vi "Default controls - save controls values.vi"(8 "error in (no error)":errorcluster) -> (0 "error out":errorcluster, 2 "VI's path in related to the INI":path, 3 "INI's path to the saved controls":path)   [LabVIEW 2020]
uses:
  Save-Load-Defaults.lvlib/Save-Load-Defaults.lvlib
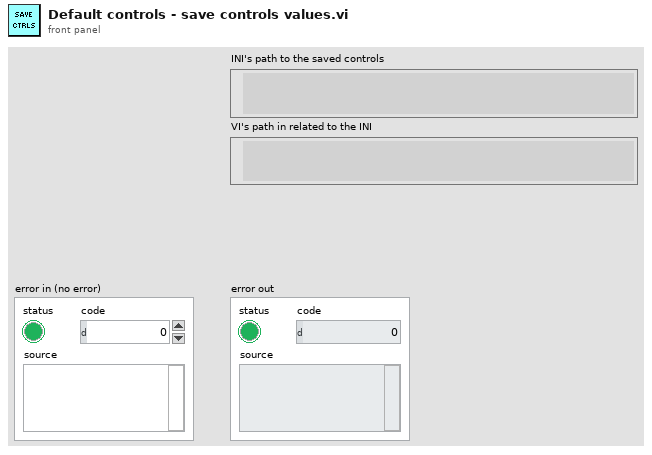
[diagram p1: front panel]
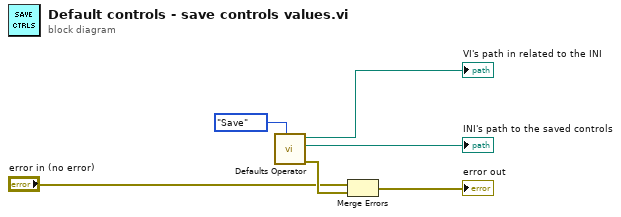
[diagram p0: block diagram]
diagram:
  n1 = call "Defaults Operator.vi"("Operation (Load)"=enum16{"Load", "Save"}."Save") -> ("error out"=w5:errorcluster, "INI's path"=→"INI's path to the saved controls":path, "VI's path"=→"VI's path in related to the INI":path)  [unwired: 8 in]
  n2 = Merge Errors("error in (no error)", w5) -> (→"error out":errorcluster)
